vi "Test Save GIF (Path).vi"(8 "error in (no error)":errorcluster) -> (0 "error out":errorcluster, 3 "Pass?":bool)   [LabVIEW 2020]
uses:
  <vilib>/picture/picture.llb/imagedata.ctl
  G-Image/G-Image.lvlib
  G-Image/Image IO/Polymorphic VIs/Load Image (Path).vi
  G-Image/Image IO/Polymorphic VIs/Save GIF Image (Path).vi
  G-Image/Image IO/Controls/Dither Type.ctl
  0f1b1910-5d7c-4507-bdef-12e0c9c3451f.vi
panel:
  out "Array":cluster{string, "new picture":picture}[](array[cluster])
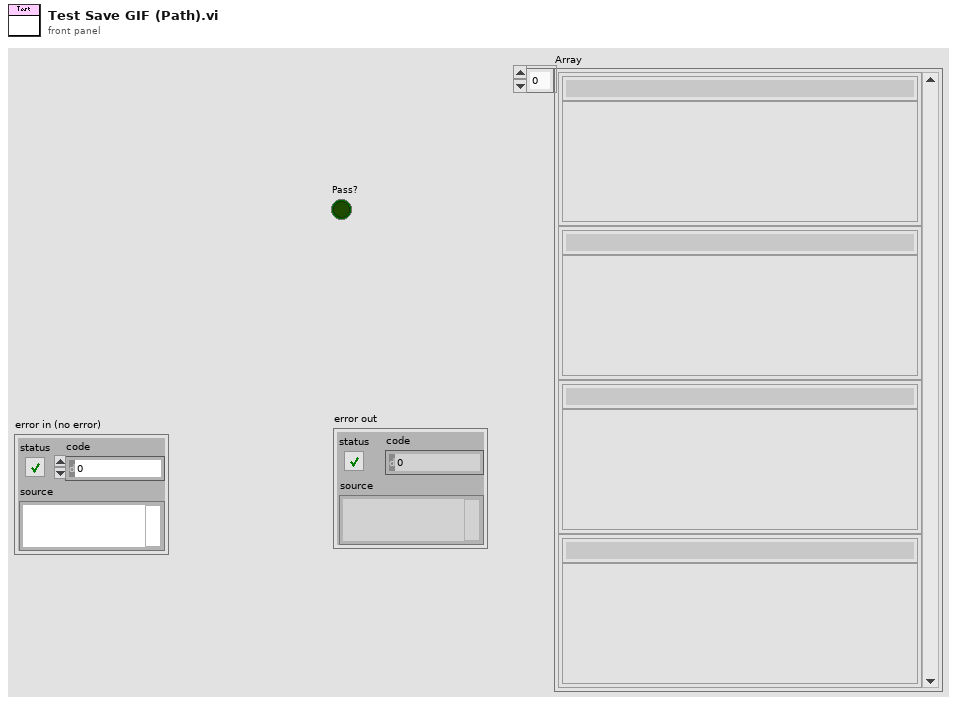
[diagram p1: front panel]
types:
  T1 = typedef "G-Image.lvlib/Dither Type.ctl" = enum32{"None", "Floyd-Steinberg"}
  T2 = typedef "imagedata.ctl" = cluster{"image type":i32, "image depth":i32, "image":u8[], "mask":u8[], "colors":u32[], "Rectangle":cluster{"left":i16, "top":i16, "right":i16, "bottom":i16}}
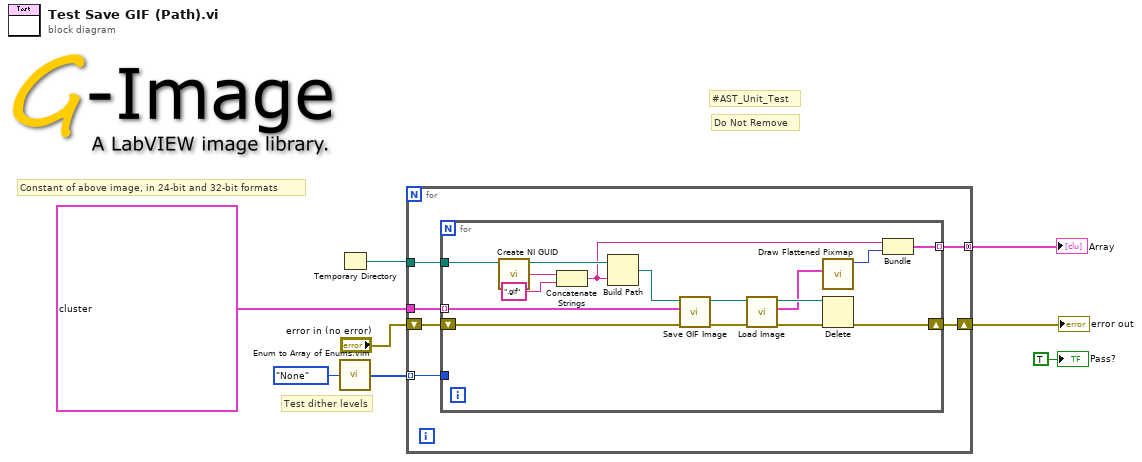
[diagram p0: block diagram]
diagram:
  # "Test dither levels"
  # "Constant of above image, in 24-bit and 32-bit formats"
  # "Do Not Remove"
  # "#AST_Unit_Test"
  n1 = Temporary Directory() -> (w7:path)
  n2 = call "Enum to Array of Enums.vim"("enum"=Dither_Type."None" ("Dither (None)")) -> ("array of enums"=w2:T1[])
  n3 = for {
    tunnel: w7 -> [w13]
    tunnel: [w12] -> w6 mode=concatenating
    tunnel: T2[] [{"image type"=0, "image depth"=24, "image"=array[115500 elements], "mask"=[], "colors"=[], "Rectangle"={"left"=0, "top"=0, "right"=350, "bottom"=110}}, {"image type"=0, "image depth"=32, "image"=array[154000 elements], "mask"=array[4840 elements], "colors"=[], "Rectangle"={"left"=0, "top"=0, "right"=350, "bottom"=110}}] ("Array 2") -> [w10]
    shift-right: [w11] -> w5
    shift-left: "error in (no error)" -> [w14]
    tunnel: w2 -> [w9] mode=indexing
    n4 = for {
      tunnel: w13 -> [w26]
      tunnel: w10 -> [w22] mode=indexing
      shift-right: [w19] -> w11
      shift-left: w14 -> [w29]
      tunnel: [w15] -> w12 mode=indexing
      tunnel: w9 -> [_]
      n5 = call <vilib>:"Create NI GUID.vi"() -> ("NI GUID"=w27:string)
      n6 = Concatenate Strings(w27, ".gif" ("string")) -> (w16:string)
      n7 = Build Path(base path=w26, name or relative path=w16) -> (appended path=w25:path)
      n8 = call-poly "Save GIF Image.vi"("error in (no error)"=w29, "Image"=w22, "Path In"=w25) -> ("error out"=w23:errorcluster, "Path Out"=w24:path)  [unwired: 7 in]
      n9 = call-poly "Load Image.vi"("error in (no error)"=w23, "Path In"=w24) -> ("error out"=w20:errorcluster, "Image"=w18:T2, "Path Out"=w21:path)  [unwired: 7 in]
      n10 = call <vilib>:"Draw Flattened Pixmap.vi"("image data"=w18) -> ("new picture"=w17:picture)  [unwired: 8 in]
      n11 = Delete(path (use dialog)=w21, error in=w20) -> (error out=w19:errorcluster)  [unwired: 3 in, 2 out]
      n12 = Bundle(w16, "new picture"=w17) -> (w15:cluster{string, "new picture":picture})  [unwired: 1 in]
    }
  }
  "error out" <- w5
  "Array" <- w6
  "Pass?" <- TRUE ("Pass?")
